vi "BinTotal.vi"(8 "error out 2":errorcluster, 9 "fileName":string="QAMT08", 10 "machine":string="QAMT08", 11 "connection reference":T1) -> (0 "error out":errorcluster, 3 "connection reference 2":T1, 4 "bin4":i32, 5 "bin2":i32, 6 "bin3":i32, 7 "bin1":i32)   [LabVIEW 2012]
uses:
  <vilib>/addons/database/Connection.llb/Conn ObjectReference.ctl
  <vilib>/addons/database/Auxilliary.llb/DB Tools Cursor Type.ctl
  <vilib>/addons/database/Connection.llb/Conn Execute.vi
  <vilib>/addons/database/Recordset.llb/Rec Fetch Integer Data (R).vi
  <vilib>/addons/database/Recordset.llb/Rec Destroy - Connection.vi
  <vilib>/addons/database/NI_Database_API.lvlib
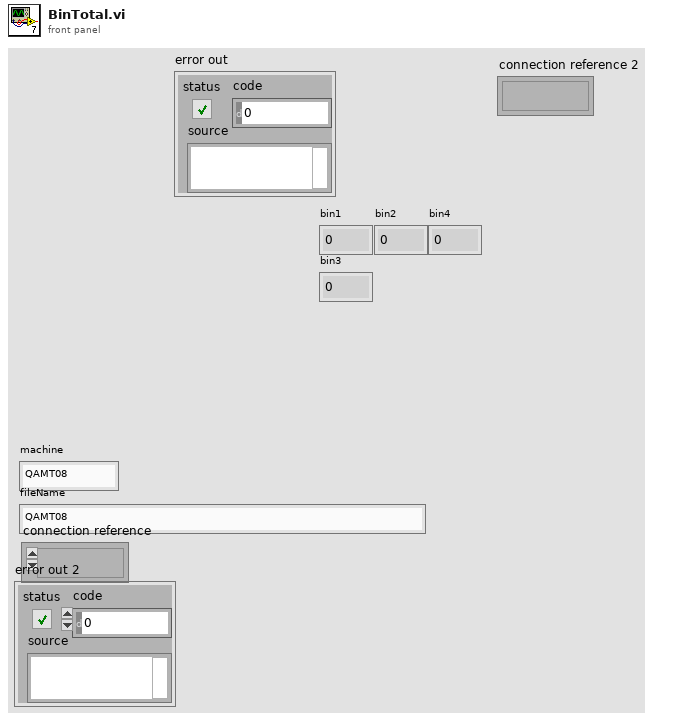
[diagram p1: front panel]
types:
  T1 = typedef "NI_Database_API.lvlib/Conn ObjectReference.ctl" = refnum<k1>
  T2 = typedef "NI_Database_API.lvlib/DB Tools Cursor Type.ctl" = enum16{"forward-only", "keyset", "dynamic", "static"}
  T3 = typedef "NI_Database_API.lvlib/Rec ObjectReference.ctl" = refnum<k1>
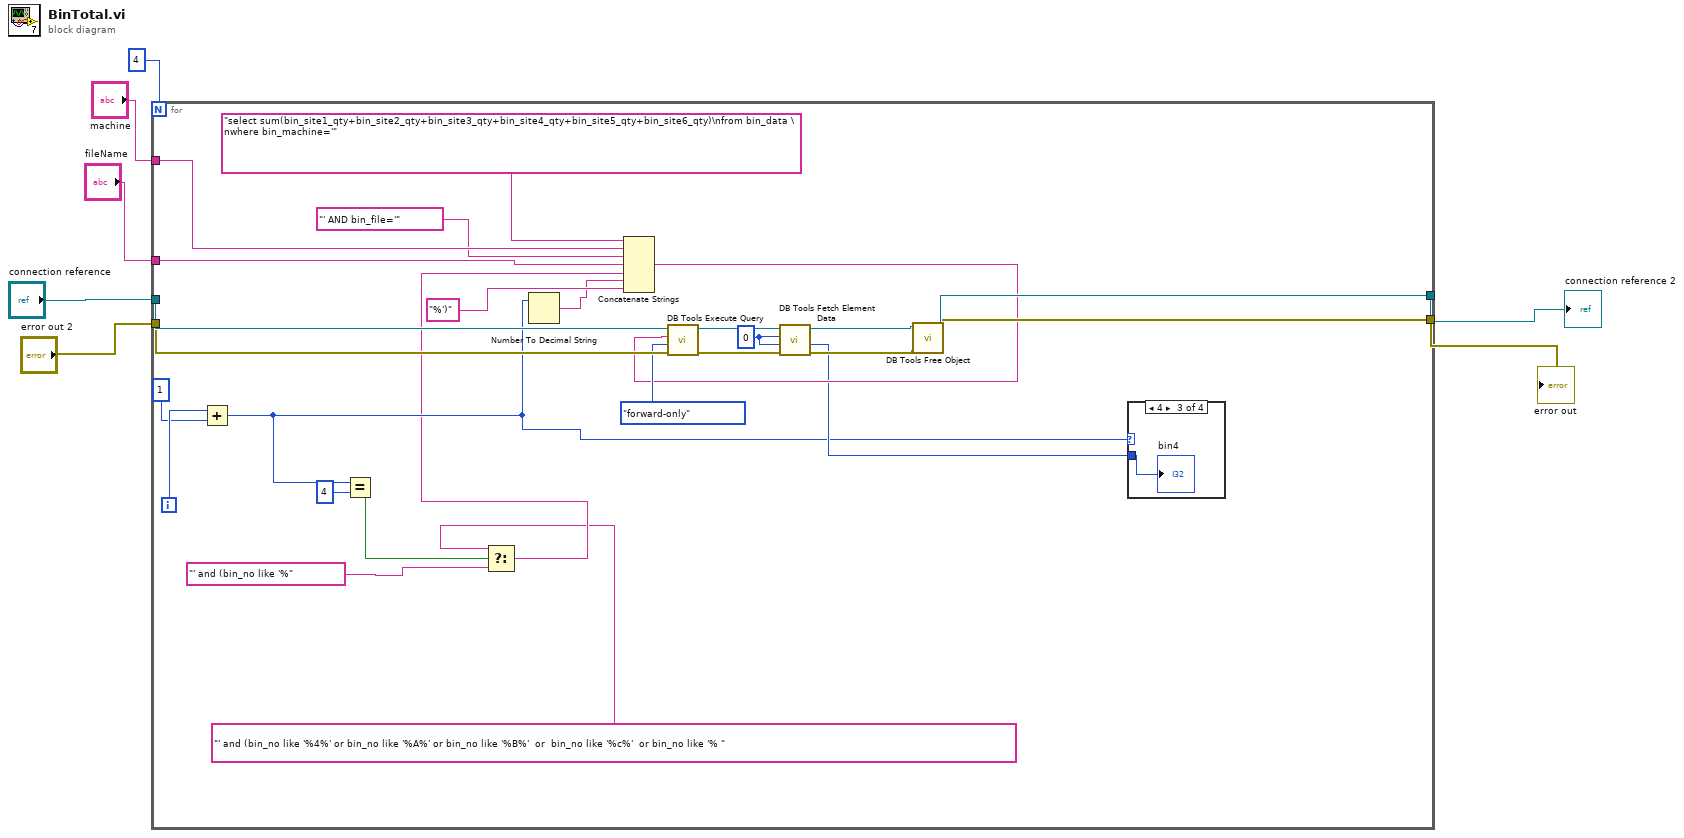
[diagram p0: block diagram]
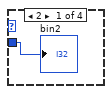
[diagram p2: hidden frame]
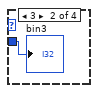
[diagram p3: hidden frame]
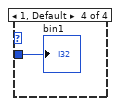
[diagram p4: hidden frame]
diagram:
  n1 = for {
    N: 4 -> [_]
    tunnel: "connection reference" -> [w33]
    tunnel: [w30] -> w3
    tunnel: "error out 2" -> [w29]
    tunnel: [w26] -> w2
    tunnel: "machine" -> [w23]
    tunnel: "fileName" -> [w21]
    i -> [w18]
    w15 = 0
    n2 = Add(x=w18, y=1) -> (x+y=w13:i32)
    n3 = Equal?(x=w13, y=4) -> (x = y?=w11:bool)
    n4 = Select(t="' and (bin_no like '%4%' or bin_no like '%A%' or bin_no like '%B%'  or  bin_no like '%c%'  or bin_no like '% " ("string"), s=w11, f="' and (bin_no like '%" ("string")) -> (s? t:f=w9:string)
    n5 = Number To Decimal String(number=w13) -> (decimal integer string=w16:string)  [unwired: 1 in]
    n6 = Concatenate Strings("select sum(bin_site1_qty+bin_site2_qty+bin_site3_qty+bin_site4_qty+bin_site5_qty+bin_site6_qty)\nfrom bin_data \nwhere bin_machine='", w23, "' AND bin_file='" ("string"), w21, w9, w16, "%')" ("string")) -> (w19:string)
    n7 = call-poly <vilib>:"DB Tools Execute Query.vi"("error in (no error)"=w29, "cursor type"=DB_Tools_Cursor_Type."forward-only", "SQL query"=w19, "connection reference"=w33) -> ("error out"=w28:errorcluster, "recordset reference"=w32:T3)  [unwired: 4 in]
    n8 = call-poly <vilib>:"DB Tools Fetch Element Data.vi"("error in (no error)"=w28, "type"=w15, "column index"=w15, "recordset reference"=w32) -> ("error out"=w27:errorcluster, "data"=w14:i32, "recordset reference out"=w31:T3)  [unwired: 3 in]
    n9 = call-poly <vilib>:"DB Tools Free Object.vi"("error in (no error)"=w27, "recordset reference"=w31) -> ("error out"=w26:errorcluster, "connection reference"=w30:T1)  [unwired: 8 in]
    n10 = case shown="4" w13 {
      tunnel: w14 -> [w34 w35 w36 w37]
      frame 2 {
        "bin2" <- w34
      }
      frame 3 {
        "bin3" <- w35
      }
      frame 4 {
        "bin4" <- w36
      }
      frame 1, Default {
        "bin1" <- w37
      }
    }
  }
  "connection reference 2" <- w3
  "error out" <- w2
